vi "控件显示.vi"(10 "Visible":bool[](array[boolean]), 11 "Ctl":refnum<vi>[](array[refnum])) -> ()   [LabVIEW 2016]
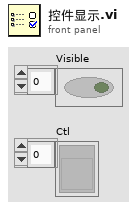
[diagram p1: front panel]
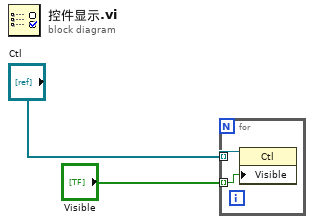
[diagram p0: block diagram]
diagram:
  n1 = for {
    tunnel: "Ctl" -> [w4] mode=indexing
    tunnel: "Visible" -> [w3] mode=indexing
    n2 = property class="Ctl"(reference=w4, "Visible"=w3) -> ()  [unwired: 1 in, 2 out]
  }
